vi "Get Delimit.vi"(8 "error in (no error)":errorcluster caption="entrée d'erreur (pas d'erreur)", 11 "Class CSV_File (Default) en entrée":refnum<class "Class CSV_File.lvclass">) -> (0 "error out":errorcluster caption="sortie d'erreur", 2 "Delimit":string, 3 "Class CSV_File (Default) en sortie":refnum<class "Class CSV_File.lvclass">)   [LabVIEW 2020, in "Library Instrument & Equipement.lvlib" / "Library File.lvlib" / "Class CSV_File.lvclass"]
uses:
  Class CSV_File.lvclass
  Class CSV_File.lvclass/Class CSV_File.ctl
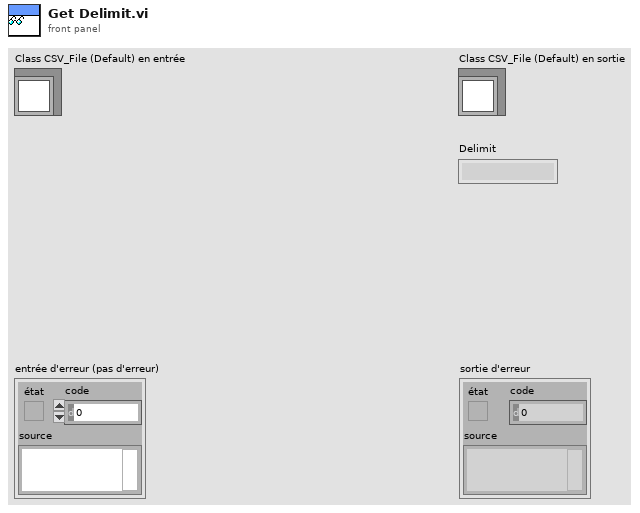
[diagram p1: front panel]
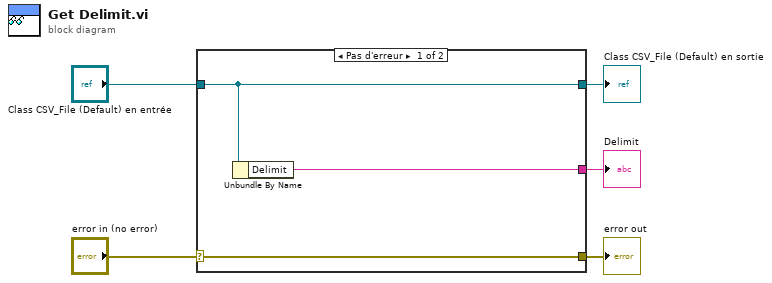
[diagram p0: block diagram]
diagram:
  n1 = case shown="Pas d'erreur" "error in (no error)" {
    selector: "error in (no error)" -> [w8 w9]
    tunnel: [w8 w9] -> w4
    tunnel: [w7 w10] -> w2
    tunnel: "Class CSV_File (Default) en entrée" -> [w7 w10]
    tunnel: [w6 _] -> w1
    frame No Error {
      n2 = Unbundle By Name(w7) -> ("Delimit"=w6:string)
    }
    frame Error {
    }
  }
  "error out" <- w4
  "Class CSV_File (Default) en sortie" <- w2
  "Delimit" <- w1
